vi "Linear Output - Adding Points (FPGA).vi"() -> ()   [LabVIEW 2017]
doc: "This VI will output a linear waveform beginning at the value in Start Point and end at the value at End Point. It will add points (values) between these two points according the the Poitns to Add (2^n-1) control.\n\nThis VI adds the points according to an algorithm that takes advantage of the binary representation of I16 interger values. This algorithm is explained on the block diagram and in the Linear Waveform Generation with CompactRIO and LabVIEW FPGA Tutorial."
uses:
  <vilib>/rvi/Emulation/niFpgaGetClockAttributes.vi
  <vilib>/rvi/Emulation/niFpgaSctlEmulationGetInTimedLoop.vi
  <vilib>/rvi/Emulation/niFpgaEmulationReportErrorSimple.vi
  <vilib>/rvi/eio/common/nirviEmuTemplateMethod_errors.vi
  <vilib>/rvi/Emulation/niFpgaCriticalErrorInLSC.vi
  <vilib>/rvi/Analysis/common/FxpNativeNode/niFpgaFxpNative.xnode
  <vilib>/eio/EIONode/EIONode.xnode
panel:
  out "rise time [uSec]":u32
  in  "Update Period (uSec)":u32=500
  in  "End Current 3":fxp<+,16,16>
  in  "Start Current 2":fxp<+,16,16>
  in  "Points to Add (2^n - 1)":i16=3
  # "* This VI will output voltages between the Start Point and End Point values.  \nThe number of points that  will be placed is determined by the Points to Add\ncontrol, and they will be output at a rate equal to 1/Update Period (mSec) \n\n* The number of points to add will equal:  2^(Points To Add) - 1;"
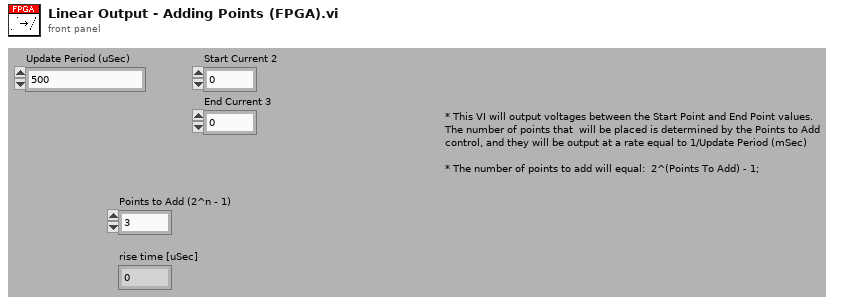
[diagram p1: front panel]
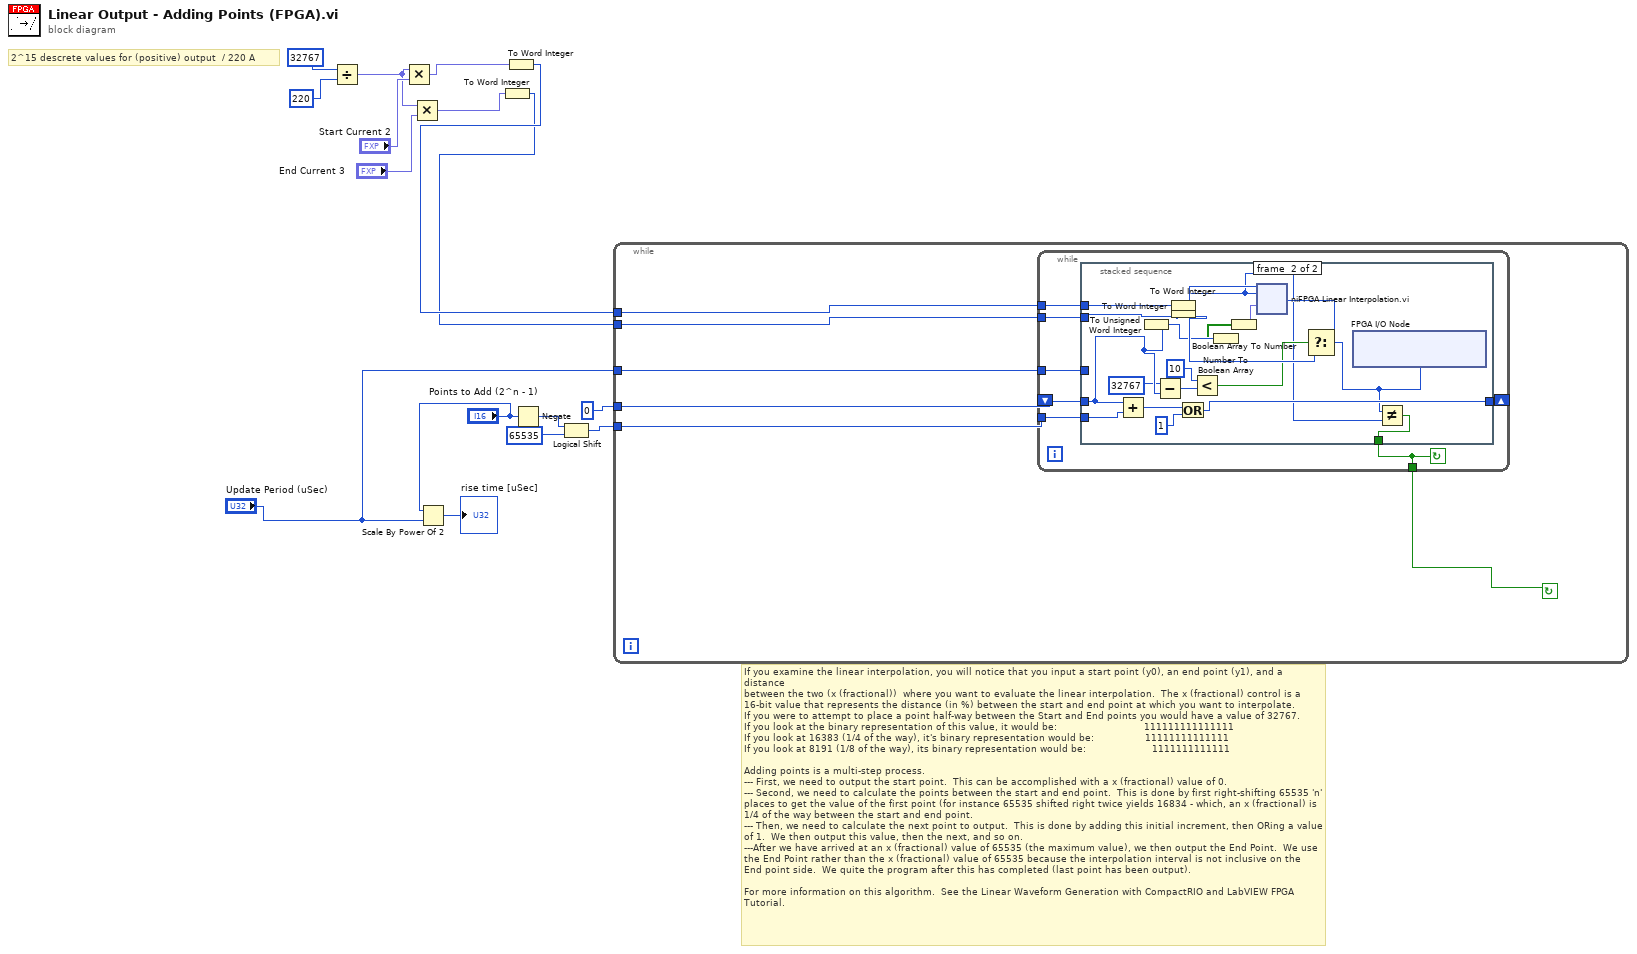
[diagram p0: block diagram]
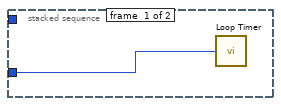
[diagram p2: hidden frame]
diagram:
  # "2^15 descrete values for (positive) output  / 220 A"
  # "If you examine the linear interpolation, you will notice that you input a start point (y0), an end point (y1), and a distance\nbetween the two (x (fractional))  where you want to evaluate the linear interpolation.  The x (fractional) control is a \n16-bit value that represents the distance (in %) between the start and end point at which you want to interpolate.  \nIf you were to attempt to place a point half-way between the Start and End points you would have a value of 32767.\nIf you look at the binary representation of this value, it would be:                             111111111111111\nIf you look at 16383 (1/4 of the way), it's binary representation would be:                 11111111111111\nIf you look at 8191 (1/8 of the way), its binary representation would be:                      1111111111111\n\nAdding points is a multi-step process.  \n--- First, we need to output the start point.  This can be accomplished with a x (fractional) value of 0.\n--- Second, we need to calculate the points between the start and end point.  This is done by first right-shifting 65535 'n' places to get the value of the first point (for instance 65535 shifted right twice yields 16834 - which, an x (fractional) is 1/4 of the way between the start and end point.\n--- Then, we need to calculate the next point to output.  This is done by adding this initial increment, then ORing a value of 1.  We then output this value, then the next, and so on.  \n---After we have arrived at an x (fractional) value of 65535 (the maximum value), we then output the End Point.  We use the End Point rather than the x (fractional) value of 65535 because the interpolation interval is not inclusive on the\nEnd point side.  We quite the program after this has completed (last point has been output).\n\nFor more information on this algorithm.  See the Linear Waveform Generation with CompactRIO and LabVIEW FPGA\nTutorial."
  n1 = Divide(x=i16 32767, y=i16 220) -> (x/y=w9:fxp<+,15,15>)
  n2 = Multiply(x=w9, y="Start Current 2") -> (x*y=w7:fxp<+,31,31>)
  n3 = Multiply(x=w9, y="End Current 3") -> (x*y=w6:fxp<+,31,31>)
  n4 = Scale By Power Of 2(n="Points to Add (2^n - 1)", x="Update Period (uSec)") -> (x*2^n=→"rise time [uSec]":u32)
  n5 = To Word Integer(number=w6) -> (16bit integer=w4:i16)
  n6 = To Word Integer(number=w7) -> (16bit integer=w5:i16)
  n7 = Negate(x="Points to Add (2^n - 1)") -> (-x=w16:i16)
  n8 = Logical Shift(y=w16, x=u16 65535) -> (x << y=w14:u16)
  n9 = while {
    tunnel: w14 -> [w22]
    tunnel: w5 -> [w21]
    tunnel: w4 -> [w20]
    tunnel: u16 0 -> [w19]
    tunnel: "Update Period (uSec)" -> [w18]
    stop <- w17 continue-if-true
    n10 = while {
      tunnel: w22 -> [w29]
      tunnel: w21 -> [w28]
      tunnel: w20 -> [w27]
      shift-right: [w26] -> _
      shift-left: w19 -> [w25]
      tunnel: w18 -> [w24]
      tunnel: [w23] -> w17
      stop <- w23 continue-if-true
      n11 = stacked-sequence {
        tunnel: w29 -> [_ w44]
        tunnel: w28 -> [_ w49]
        tunnel: w27 -> [_ w47]
        tunnel: [_ w33] -> w23
        tunnel: [_ w43] -> w26
        tunnel: w25 -> [_ w38]
        tunnel: w24 -> [w30 _]
        frame #0 {
          n12 = call "Loop Timer"("Count(uSec)"=w30) -> ()  [unwired: 1 out]
        }
        frame #1 {
          n13 = Add(x=w38, y=w44) -> (x+y=w46:u16)
          n14 = To Unsigned Word Integer(number=w38) -> (unsigned 16bit integer=w42:u16)
          n15 = Subtract(x=u16 32767 ("y"), y=w38) -> (x-y=w35:u16)
          n16 = To Word Integer(number=w49) -> (16bit integer=w39:i16)
          n17 = To Word Integer(number=w47) -> (16bit integer=w31:i16)
          n18 = Or(x=w46, y=u16 1) -> (x .or. y?=w43:u16)
          n19 = Less?(x=i16 10, y=w35) -> (x < y?=w36:bool)
          n20 = Number To Boolean Array(number=w42) -> (Boolean array=w40:bool[])
          n21 = Boolean Array To Number(Boolean array=w40) -> (number=w41:fxp<+,15,0>)
          n22 = xnode ("niFPGA Linear Interpolation.vi")("y0"=w39, "y1"=w31, "x"=w41) -> ("y"=w48:i16)
          n23 = Select(t=w48, s=w36, f=w47) -> (s? t:f=w32:i16)
          n24 = xnode "FPGA I/O Node"("Connector0/AO0"=w32) -> ()  [unwired: 1 in, 1 out]
          n25 = Not Equal?(x=w32, y=w31) -> (x != y?=w33:bool)
        }
      }
    }
  }
